vi "VS_RunStimulusProfile.vi"(0 "Engine Reference(in)":refnum<k7>, 1 "Condition Run?":bool, 2 "Working Directory":string, 3 "Stim Profile path":string, 5 "Sequence File Ref(in)":refnum<k7>, 7 "VeriStand version info":T1, 9 "Stim profile":string, 11 "error in":errorcluster, 12 "Step Group":i32(ring) items=["StepGroup_Setup", "StepGroup_Main", "StepGroup_Cleanup"], 13 "Step Index":i32, 14 "Requirement":string) -> (4 "Engine reference(out)":refnum<k7>, 6 "Sequence File Ref(out)":refnum<k7>, 8 "VeriStand version info (out)":T1, 10 "VS Log file":string, 15 "error out":errorcluster)   [LabVIEW 2010]
doc: "This VI creates a TestStand step that runs a VeriStand Stimulus Profile and logs data in the \"Working Directory/VS Logs\" folder. If folder doesn't exist, the VI will create it."
uses:
  Ctls/dotNetAssemblyInfo.ctl
  Ctls/VSModuleTokens.ctl
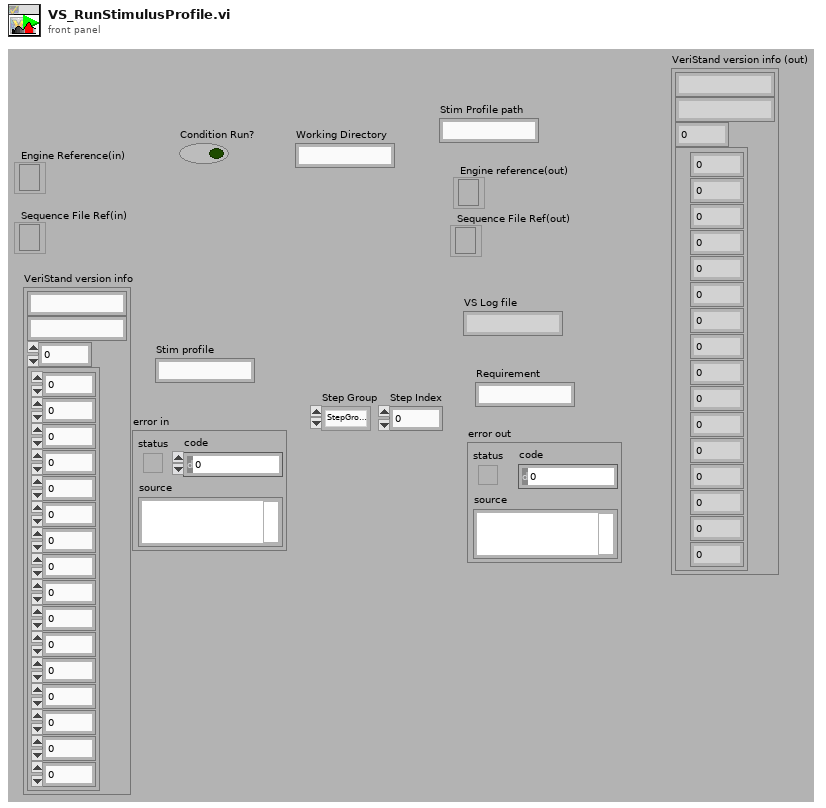
[diagram p1: front panel]
types:
  T1 = typedef "dotNetAssemblyInfo.ctl" = cluster{"VeriStand.exe Path":string, "Assembly":string, "Constructor Token":i32, "Module Token":T2}
  T2 = typedef "VSModuleTokens.ctl" = cluster{"GetIWorkspaceToken":i32, "GetIStimulusToken":i32, "GetIModelManagerToken":i32, "GetIProjectToken":i32, "RunProjectToken":i32, "CloseProjectToken":i32, "RunWorkspaceToken":i32, "StopWorkspaceToken":i32, "SetSingleChannelToken":i32, "SetMultipleParametersToken":i32, "RunStimulusToken":i32, "GetStimulusStateToken":i32, "Open WorkspaceToken":i32, "DeployToken":i32, "UndeployToken":i32, "QuitToken":i32}
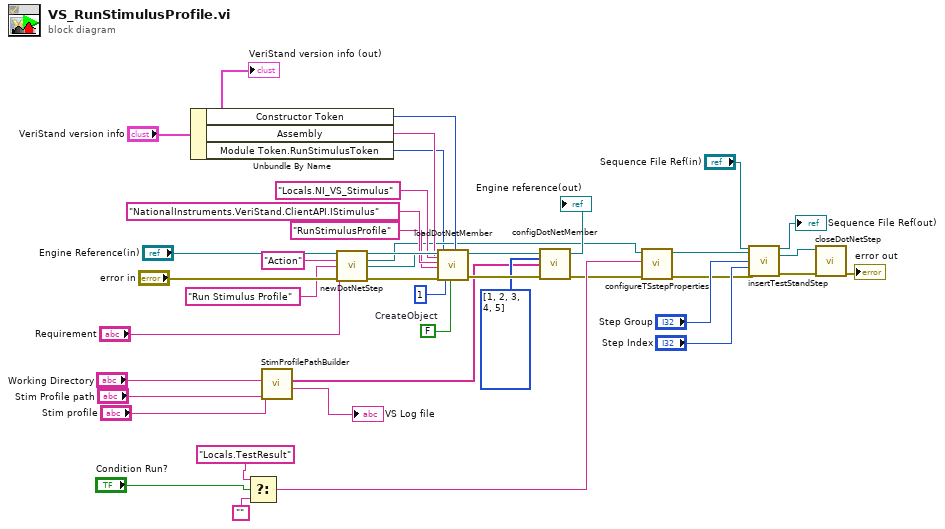
[diagram p0: block diagram]
diagram:
  w24 = FALSE  # CreateObject
  n1 = Unbundle By Name("VeriStand version info") -> ("Constructor Token"=w18:i32, "Assembly"=w19:string, "Module Token.RunStimulusToken"=w7:i32)
  n2 = Select(t="Locals.TestResult", s="Condition Run?", f="") -> (s? t:f=w10:string)
  n3 = call "StimProfilePathBuilder.vi"("Stim profile path"="Stim Profile path", "Stim profile"="Stim profile", "Working Directory"="Working Directory") -> ("VS Log file"=→"VS Log file":string, "Stim Parameters"=w6:string[])  [unwired: 7 in]
  n4 = call "newDotNetStep.vi"("Engine reference"="Engine Reference(in)", "stepType"="Action", "Step Name"="Run Stimulus Profile", "Requirement"="Requirement", "error in"="error in") -> ("Engine reference(out)"=→"Engine reference(out)":refnum<k7>, "NewStep (out)"=w12:refnum<k7>, "dotNetModule(out)"=w28:refnum<k7>, "error out"=w40:errorcluster)  [unwired: 7 in]
  n5 = call "loadDotNetMember.vi"("dotNetModule"=w28, "Strong Assembly path"=w19, "ClassName"="NationalInstruments.VeriStand.ClientAPI.IStimulus", "MemberName"="RunStimulusProfile", "Member token"=w7, "error in(no error)"=w40, "ClassReference"="Locals.NI_VS_Stimulus", "Call Member?"=1 ("Call Memeber?"), "CreateObject"=w24, "Constructor Token"=w18) -> ("dotNetModule(out)"=w23:refnum<k7>, "error out"=w22:errorcluster)  [unwired: 8 in]
  n6 = call "configDotNetMember.vi"("dotNetModule"=w23, "Index array"=i32[] [1, 2, 3, 4, 5], "Parameter Value array"=w6, "error in (no error)"=w22) -> ("error out"=w9:errorcluster)  [unwired: 11 in]
  n7 = call "configureTSstepProperties.vi"("error in"=w9, "Precondition"=w10, "NewStep (in)"=w12) -> ("error out"=w8:errorcluster, "NewStep (out)"=w11:refnum<k7>)  [unwired: 7 in]
  n8 = call "insertTestStandStep.vi"("Sequence File Ref"="Sequence File Ref(in)", "Step to insert"=w11, "Step Group"="Step Group", "index"="Step Index", "error out"=w8) -> ("Sequence File Ref(out)"=→"Sequence File Ref(out)":refnum<k7>, "Step to insert (out)"=w39:refnum<k7>, "error out"=w37:errorcluster)  [unwired: 8 in]
  n9 = call "closeDotNetStep.vi"("error in"=w37, "NewStep"=w39) -> ("error out"=→"error out":errorcluster)  [unwired: 9 in]
  "VeriStand version info (out)" <- "VeriStand version info"
